vi "From LabVIEW.vi"(4 "AlbumMap in":refnum<class "VehicleMap.lvclass">, 8 "error in (no error)":errorcluster, 10 "Value":refnum<class>) -> (0 "error out":errorcluster, 2 "DbRow":variant)   [LabVIEW 2020, in "VehicleMap.lvclass"]
uses:
  VehicleMap.lvclass
  C:/Program Files/National Instruments/LabVIEW 2024/vi.lib/Viviota/shared/ORM.lvlibp/ORM/TypeMap/TypeMap.lvclass
  Vehicle/Vehicle.lvclass
  Vehicle/Vehicle.lvclass/Vehicle.ctl
  Vehicle/Read Make.vi
  Vehicle/Read Model.vi
  Vehicle/Read Year.vi
  Vehicle/Read VehicleID.vi
  <vilib>/Viviota/shared/ORM.lvlibp/ORM/TypeMap/Read Autokey.vi
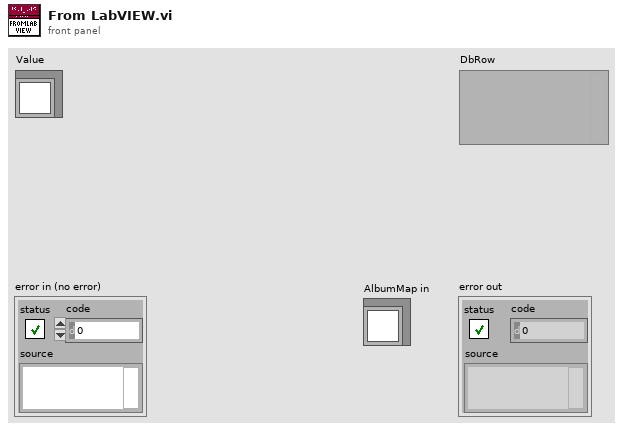
[diagram p1: front panel]
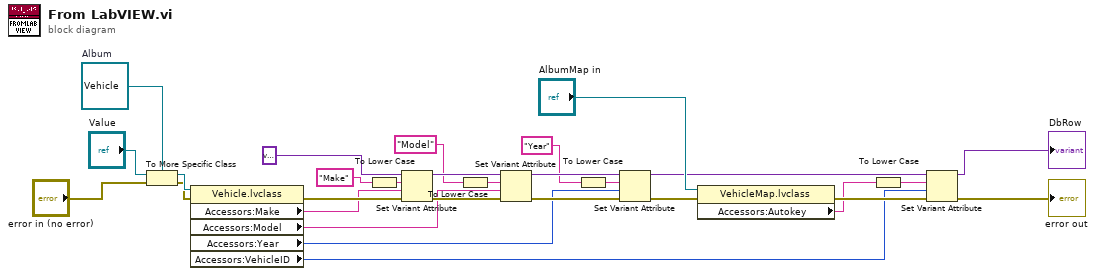
[diagram p0: block diagram]
diagram:
  w27 = refnum<class "Vehicle.lvclass"> refnum  # Album
  n1 = To More Specific Class(target class=w27, reference="Value", error in="error in (no error)") -> (specific class reference=w26:refnum<class "Vehicle.lvclass">, error out=w25:errorcluster)
  n2 = property class="Vehicle.lvclass"(reference=w26, error in=w25) -> (error out=w29:errorcluster, "Accessors:Make"=w17:string, "Accessors:Model"=w16:string, "Accessors:Year"=w15:i32, "Accessors:VehicleID"=w8:i32)  [unwired: 1 out]
  n3 = To Lower Case(string="Make" ("name")) -> (all lower case string=w4:string)
  n4 = Set Variant Attribute(Variant=variant, name=w4, value=w17, error in=w29) -> (Variant out=w21:variant, error out=w20:errorcluster)  [unwired: 1 out]
  n5 = To Lower Case(string="Model" ("name")) -> (all lower case string=w3:string)
  n6 = Set Variant Attribute(Variant=w21, name=w3, value=w16, error in=w20) -> (Variant out=w19:variant, error out=w18:errorcluster)  [unwired: 1 out]
  n7 = To Lower Case(string="Year" ("name")) -> (all lower case string=w2:string)
  n8 = Set Variant Attribute(Variant=w19, name=w2, value=w15, error in=w18) -> (Variant out=w11:variant, error out=w14:errorcluster)  [unwired: 1 out]
  n9 = property class="VehicleMap.lvclass"(reference="AlbumMap in", error in=w14) -> (error out=w13:errorcluster, "Accessors:Autokey"=w9:string)  [unwired: 1 out]
  n10 = To Lower Case(string=w9) -> (all lower case string=w1:string)
  n11 = Set Variant Attribute(Variant=w11, name=w1, value=w8, error in=w13) -> (Variant out=→"DbRow":variant, error out=→"error out":errorcluster)  [unwired: 1 out]
